vi "Open Cal Data Session.vi"(0 "fpga reference":refnum<k20>, 11 "error in":errorcluster, 12 "emulation model name":T1) -> (4 "session out":refnum<class "niHSAI Cal Data v1 Host.lvclass">, 15 "error out":errorcluster)   [LabVIEW 2021, in "Device Session.lvclass"]
doc: "Reads calibration data from the device and creates a Calibration Data session to allow you to access this data.\n\n<B>Input Parameters</B>\n\n<B>fpga reference</B> specifies a reference to the FPGA target to read calibration data from.\n\n<B>error in</B> describes error conditions that occur before this node runs. This input provides standard error in functionality.\n\n<B>emulation model name</B> specifies the model to emulate, if the 'fpga reference' is opened in a simulated or emulated context.\n\n<B>Output Parameters</B>\n\n<B>session out</B> passes a reference to your session to the next VI. 'session out' is obtained from the 'Open Session' VI of the Configuration library.\n\n<B>error out</B> contains error information. This output provides standard error out functionality."
uses:
  Device Session.lvclass
  <instrlib>/HSAI-RIO/Cal Data/Interface/v1/Host/Cal Data/niHSAI Cal Data v1 Host.lvclass
  <instrlib>/HSAI-RIO/Types/v1/Host/Typedefs/Model Name.ctl
  <instrlib>/HSAI-RIO/Cal Data/Group A/v1/Host/Cal Data/niHSAI Group A Cal Data v1 Host.lvclass
  C:/Program Files (x86)/National Instruments/LabVIEW 2021/instr.lib/HSAI-RIO/Cal Data/Group A Base/v1/Host/Cal Data/niHSAI Group A Base Cal Data v1 Host.lvclass
  <instrlib>/HSAI-RIO/Cal Data/Group A1/v1/Host/Cal Data/niHSAI Group A1 Cal Data v1 Host.lvclass
  <instrlib>/HSAI-RIO/Cal Data/Group A Base/v1/Host/Cal Data/niHSAI Group A Base Cal Data v1 Host.lvclass
  C:/Program Files (x86)/National Instruments/LabVIEW 2021/instr.lib/HSAI-RIO/Cal Data/Interface/v1/Host/Cal Data/niHSAI Cal Data v1 Host.lvclass
  <vilib>/Utility/error.llb/Error Cluster From Error Code.vi
  <vilib>/ErrorRing/Error Ring.xnode
  <instrlib>/HSAI-RIO/Utilities/v1/Host/niHSAI Utilities v1 Host.lvlib
  <vilib>/LabVIEW Targets/FPGA/Digitizers/Plugin Interface/niHSAI Plugin Interface.lvlib
  <instrlib>/HSAI-RIO/Config/Common/niHSAI Common Config v1 Host.lvlib
  <instrlib>/HSAI-RIO/Types/v1/Host/niHSAI Types v1 Host.lvlib
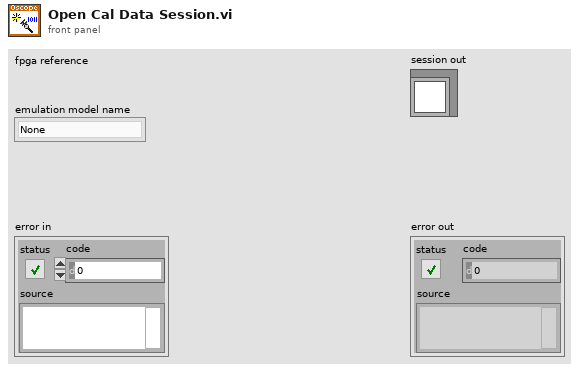
[diagram p1: front panel]
types:
  T1 = typedef "niHSAI Types v1 Host.lvlib/Model Name.ctl" = enum8{"None", "PXIe-5170R (4CH)", "PXIe-5170R (8CH)", "PXIe-5171R (8CH)", "PXIe-5172 (4CH - 325T)", "PXIe-5172 (8CH - 325T)", "PXIe-5172 (8CH - 410T)", "PXIe-5164", "PXIe-5163"}
  T2 = typedef "niHSAI Types v1 Host.lvlib/Product Info.ctl" = cluster{"product ID":u32, "device group":T3, "model name":T1}
  T3 = typedef "niHSAI Types v1 Host.lvlib/Device Group.ctl" = enum16{"Undefined", "Group A", "Group B"}
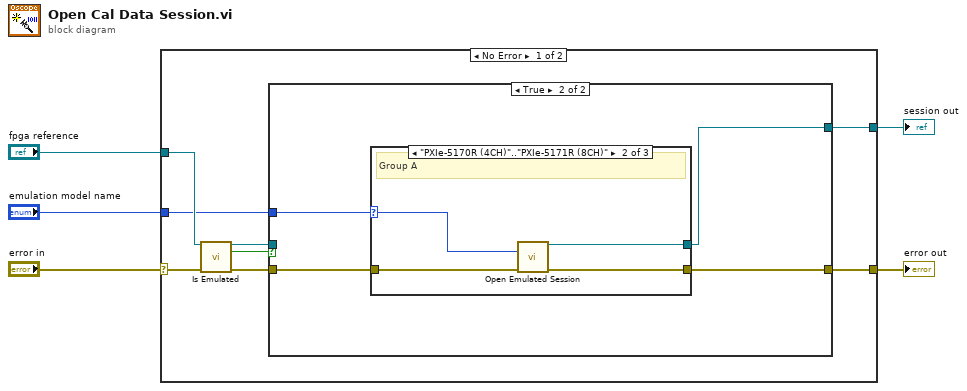
[diagram p0: block diagram]
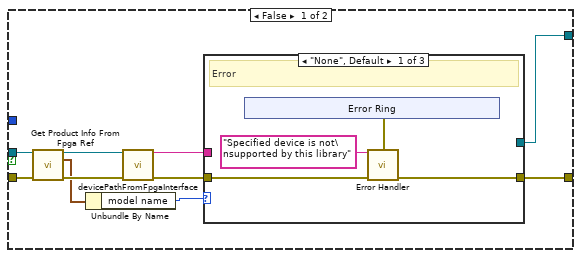
[diagram p2: hidden frame]
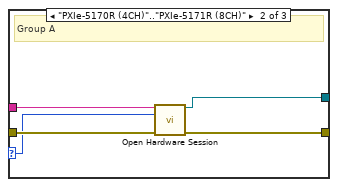
[diagram p3: hidden frame]
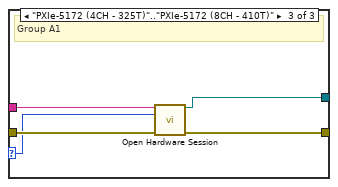
[diagram p4: hidden frame]
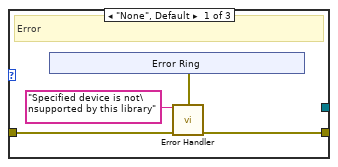
[diagram p5: hidden frame]
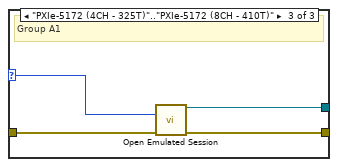
[diagram p6: hidden frame]
diagram:
  n1 = case shown="No Error" "error in" {
    selector: "error in" -> [w13 w62]
    tunnel: [w8 w62] -> w2
    tunnel: "fpga reference" -> [w12 _]
    tunnel: [w7 _] -> w1
    tunnel: "emulation model name" -> [w6 _]
    frame No Error {
      n2 = call <instrlib>:"Is Emulated.vi"("fpga interface in"=w12, "error in"=w13) -> ("fpga interface out"=w10:refnum<k20>, "is emulated?"=w11:bool, "error out"=w9:errorcluster)  [unwired: 10 in, 1 out]
      n3 = case shown="True" w11 {
        tunnel: w10 -> [w21 _]
        tunnel: w9 -> [w22 w45]
        tunnel: [w14 w44] -> w8
        tunnel: [w15 w43] -> w7
        tunnel: w6 -> [_ w42]
        frame False {
          n4 = call <instrlib>:"Get Product Info From Fpga Ref.vi"("fpga interface in"=w21, "error in"=w22) -> ("fpga interface out"=w20:refnum<k20>, "product info"=w19:T2, "error out"=w23:errorcluster)  [unwired: 11 in]
          n5 = Unbundle By Name(w19) -> ("model name"=w16:T1)
          n6 = call <vilib>:"devicePathFromFpgaInterface.vi"("fpga interface"=w20, "error in"=w23) -> ("device path"=w17:string, "error out"=w18:errorcluster)  [unwired: 12 in]
          n7 = case shown="\"None\", Default" w16 {
            selector: w16 -> [_ w32 w38]
            tunnel: [w25 w36 w41] -> w14
            tunnel: [_ w35 w37] -> w15
            tunnel: w17 -> [_ w34 w40]
            tunnel: w18 -> [w26 w33 w39]
            frame "None", Default {
              # "Error"
              n8 = xnode "Error Ring"() -> ("error out"=w27:errorcluster)
              n9 = call <instrlib>:"Error Handler.vi"("error message (\"\")"="Specified device is not\nsupported by this library", "new error in"=w27, "error in"=w26) -> ("error out"=w25:errorcluster)  [unwired: 12 in]
            }
            frame "PXIe-5170R (4CH)".."PXIe-5171R (8CH)" {
              # "Group A"
              n10 = call <instrlib>:"Open Hardware Session.vi"("device path"=w34, "model name"=w32, "error in"=w33) -> ("calibration data out"=w35:refnum<class "niHSAI Group A Cal Data v1 Host.lvclass">, "error out"=w36:errorcluster)  [unwired: 11 in]
            }
            frame "PXIe-5172 (4CH - 325T)".."PXIe-5172 (8CH - 410T)" {
              # "Group A1"
              n11 = call <instrlib>:"Open Hardware Session.vi"("device path"=w40, "model name"=w38, "error in"=w39) -> ("calibration data out"=w37:refnum<class "niHSAI Group A1 Cal Data v1 Host.lvclass">, "error out"=w41:errorcluster)  [unwired: 11 in]
            }
          }
        }
        frame True {
          n12 = case shown="\"PXIe-5170R (4CH)\"..\"PXIe-5171R (8CH)\"" w42 {
            selector: w42 -> [_ w55 w58]
            tunnel: [w47 w57 w60] -> w44
            tunnel: [_ w54 w59] -> w43
            tunnel: w45 -> [w48 w56 w61]
            frame "None", Default {
              # "Error"
              n13 = xnode "Error Ring"() -> ("error out"=w49:errorcluster)
              n14 = call <instrlib>:"Error Handler.vi"("error message (\"\")"="Specified device is not\nsupported by this library", "new error in"=w49, "error in"=w48) -> ("error out"=w47:errorcluster)  [unwired: 12 in]
            }
            frame "PXIe-5170R (4CH)".."PXIe-5171R (8CH)" {
              # "Group A"
              n15 = call <instrlib>:"Open Emulated Session.vi"("model name"=w55, "error in"=w56) -> ("calibration data out"=w54:refnum<class "niHSAI Group A Cal Data v1 Host.lvclass">, "error out"=w57:errorcluster)  [unwired: 12 in]
            }
            frame "PXIe-5172 (4CH - 325T)".."PXIe-5172 (8CH - 410T)" {
              # "Group A1"
              n16 = call <instrlib>:"Open Emulated Session.vi"("model name"=w58, "error in"=w61) -> ("calibration data out"=w59:refnum<class "niHSAI Group A1 Cal Data v1 Host.lvclass">, "error out"=w60:errorcluster)  [unwired: 12 in]
            }
          }
        }
      }
    }
    frame Error {
    }
  }
  "session out" <- w1
  "error out" <- w2
